vi "Panel to Terminal Configs.vi"(11 "Panels":refnum<class "ArrayPanel.lvclass">[](array[class])) -> (3 "Terminal Configs":T1[](array[typedef]))   [LabVIEW 2020, in "FlexBlocks.lvlib"]
uses:
  FlexBlocks.lvlib
  Value Editor Base/Value Editor Base.lvclass
  Terminal Direction.ctl
  Value Mode.ctl
  Special Terminal.ctl
  Type Descriptor.ctl
  Terminal Mode.ctl
  Terminal Config.ctl
  <vilib>/IlluminatedG/IG OOPanel/OOPanel/ArrayPanel/ArrayPanel.lvclass
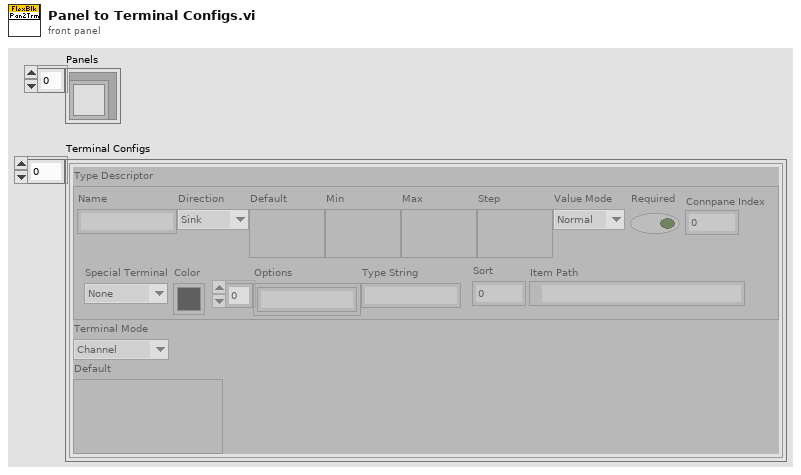
[diagram p1: front panel]
types:
  T1 = typedef "FlexBlocks.lvlib/Terminal Config.ctl" = cluster{"Type Descriptor":T2, "Terminal Mode":T6, "Default":variant}
  T2 = typedef "FlexBlocks.lvlib/Type Descriptor.ctl" = cluster{"Name":string, "Direction":T3, "Default":variant, "Min":variant, "Max":variant, "Step":variant, "Value Mode":T4, "Required":bool, "Connpane Index":i32, "Special Terminal":T5, "Color":u32, "Options":string[], "Type String":string, "Sort":i32, "Item Path":path}
  T3 = typedef "FlexBlocks.lvlib/Terminal Direction.ctl" = enum16{"Sink", "Source"}
  T4 = typedef "FlexBlocks.lvlib/Value Mode.ctl" = enum16{"Normal", "Range", "Select"}
  T5 = typedef "FlexBlocks.lvlib/Special Terminal.ctl" = enum16{"None", "Action", "Init", "Tag", "State in", "State out", "Error"}
  T6 = typedef "FlexBlocks.lvlib/Terminal Mode.ctl" = enum16{"Channel", "Config", "Value", "Control Ref"}
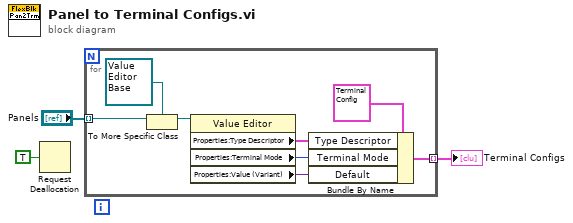
[diagram p0: block diagram]
diagram:
  n1 = Request Deallocation(TRUE ("flag")) -> ()
  n2 = for {
    tunnel: "Panels" -> [w11] mode=indexing
    tunnel: [w4] -> w2 mode=indexing
    n3 = To More Specific Class(target class=refnum<class "Value Editor Base.lvclass"> refnum ("FlexBlocks.lvlib:Value Editor Base.lvclass"), reference=w11) -> (specific class reference=w9:refnum<class "Value Editor Base.lvclass">)  [unwired: 1 in, 1 out]
    n4 = property class="Value Editor"(reference=w9) -> ("Properties:Type Descriptor"=w7:T2, "Properties:Terminal Mode"=w6:T6, "Properties:Value (Variant)"=w5:variant)  [unwired: 1 in, 2 out]
    n5 = Bundle By Name(cluster=T1 {"Type Descriptor"={"Name"="", "Direction"=enum."Sink", "Default"=variant, "Min"=variant, "Max"=variant, "Step"=variant, "Value Mode"=enum."Normal", "Required"=FALSE, "Connpane Index"=0, "Special Terminal"=enum."None", "Color"=0, "Options"=[], "Type String"="", "Sort"=0, "Item Path"=path ""}, "Terminal Mode"=enum."Channel", "Default"=variant} ("Terminal Config"), "Type Descriptor"=w7, "Terminal Mode"=w6, "Default"=w5) -> (w4:T1)
  }
  "Terminal Configs" <- w2
